vi "write_log_camera.vi"(8 "error in (no error)":errorcluster, 10 "Cluster 2":T1, 11 "Log File in":refnum<k34>) -> (0 "error out":errorcluster, 3 "Log File out":refnum<k34>)   [LabVIEW 2017]
uses:
  Control 2.ctl
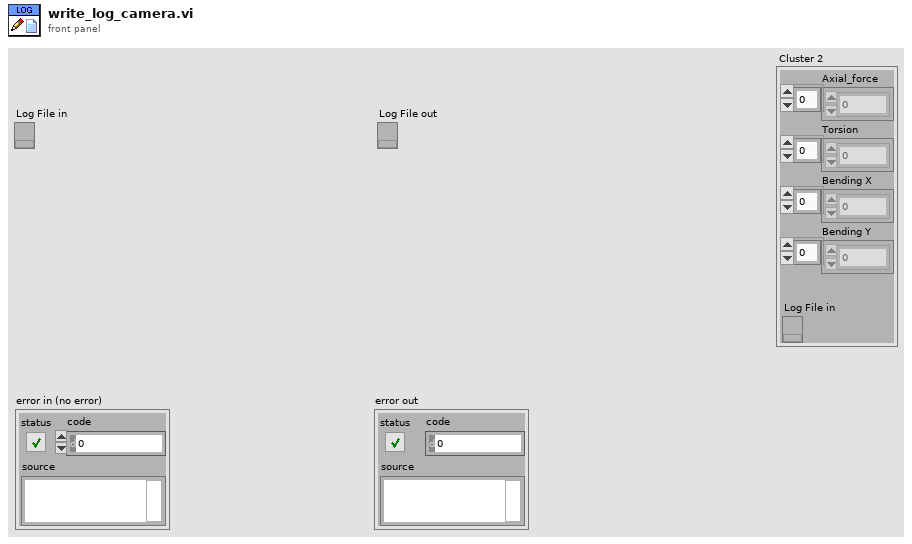
[diagram p1: front panel]
types:
  T1 = typedef "Control 2.ctl" = cluster{"Axial_force":i16[], "Torsion":i16[], "Bending X":i16[], "Bending Y":i16[], "Log File in":refnum<k34>}
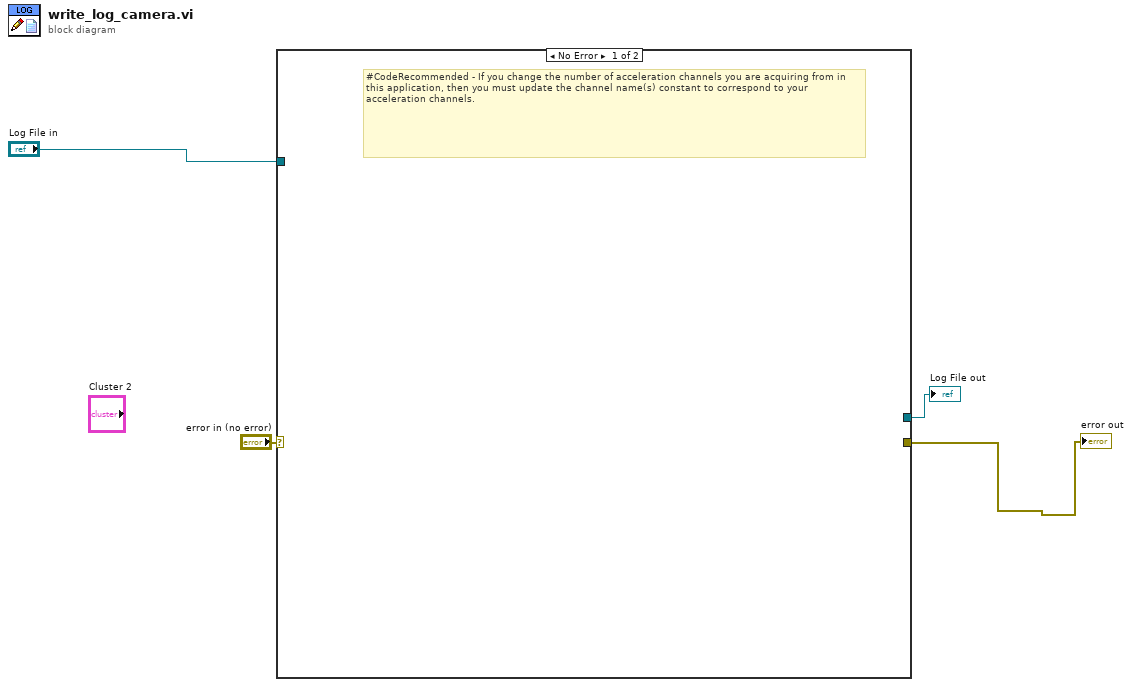
[diagram p0: block diagram]
diagram:
  n1 = case shown="No Error" "error in (no error)" {
    selector: "error in (no error)" -> [_ w5]
    tunnel: "Log File in" -> [_ w6]
    tunnel: [_ w6] -> w3
    tunnel: [_ w5] -> w1
    frame No Error {
      # "#CodeRecommended - If you change the number of acceleration channels you are acquiring from in this application, then you must update the channel name(s) constant to correspond to your acceleration channels."
    }
    frame Error {
    }
  }
  "Log File out" <- w3
  "error out" <- w1
